vi "JSON Path from ID and item List.vi"(8 "error in (no error)":errorcluster, 10 "Item List":string[](array[string]), 11 "Item ID":string) -> (0 "error out":errorcluster, 2 "Item JSON string":string)   [LabVIEW 2020, in "JSON File Manipulation.lvlib"]
doc: "Outputs the JSON string for the object referenced by the Item ID input from the JSON object list. Returns an error if the item ID is not valid or does not exist."
uses:
  JSON File Manipulation.lvlib
  <vilib>/Utility/error.llb/Error Cluster From Error Code.vi
  <vilib>/ErrorRing/Error Ring.xnode
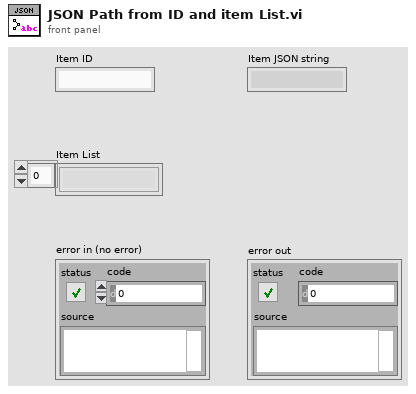
[diagram p1: front panel]
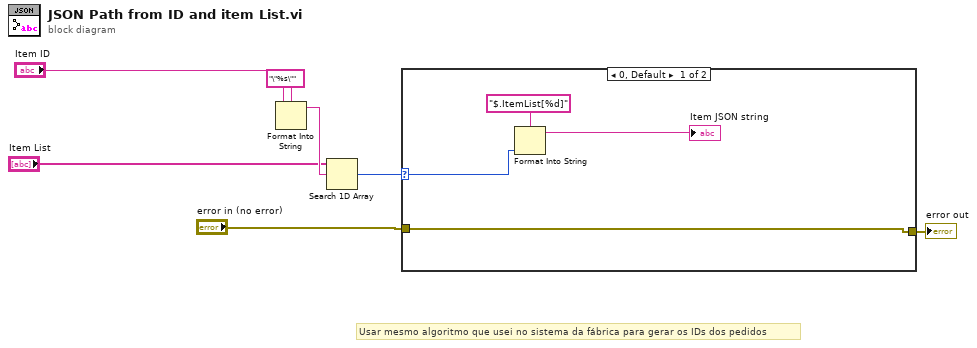
[diagram p0: block diagram]
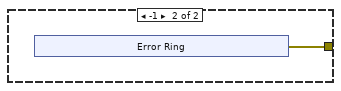
[diagram p2: hidden frame]
diagram:
  # "Usar mesmo algoritmo que usei no sistema da fábrica para gerar os IDs dos pedidos"
  n1 = Format Into String(format string="\"%s\"", "Item ID") -> (resulting string=w4:string)  [unwired: 2 in, 1 out]
  n2 = Search 1D Array(1D array="Item List", element=w4) -> (index of element=w6:i32)  [unwired: 1 in]
  n3 = case shown="0, Default" w6 {
    selector: w6 -> [w9 _]
    tunnel: [w8 w12] -> w2
    tunnel: "error in (no error)" -> [w8 _]
    frame 0, Default {
      n4 = Format Into String(format string="$.ItemList[%d]" ("$Path or Item Name"), w9) -> (resulting string=→"Item JSON string":string)  [unwired: 2 in, 1 out]
    }
    frame -1 {
      n5 = xnode "Error Ring"() -> ("error out"=w12:errorcluster)
    }
  }
  "error out" <- w2
